vi "Valid Resource.vi"(8 "error in (no error)":errorcluster, 10 "RP2040.lvlib:VisaResource":refnum<class "VisaResource.lvclass">) -> (0 "error out":errorcluster, 2 "Valid?":bool)   [LabVIEW 2020, in "RP2040.lvlib" / "RP2040Platform.lvclass"]
uses:
  RP2040Platform.lvclass
  Builds/picoG/ppl/PicoG-Core.lvlibp/PicoG-Processor/PicoG-Core/VisaResource/VisaResource.lvclass
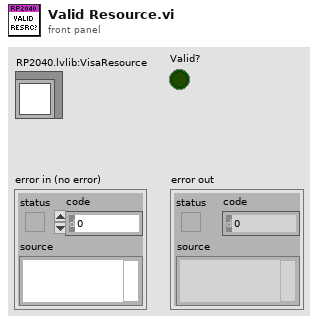
[diagram p1: front panel]
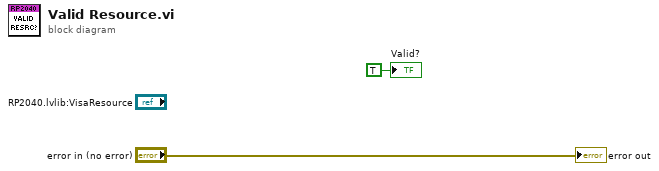
[diagram p0: block diagram]
diagram:
  "error out" <- "error in (no error)"
  "Valid?" <- TRUE ("Valid?")
